vi "Ex2_Adquiere_Datos.vi"(8 "error in (no error)":errorcluster, 11 "LINX Resource in":T2) -> (0 "error out":errorcluster, 2 "Señales":T1, 3 "LINX Resource out":T2)   [LabVIEW 2020]
uses:
  <vilib>/MakerHub/LINX/Private/Type Defs/LINX Ref.ctl
  <vilib>/MakerHub/LINX/Private/Type Defs/Platform.ctl
  <vilib>/MakerHub/LINX/Private/Type Defs/Interface.ctl
  <vilib>/MakerHub/LINX/Private/Device/Type Defs/LINX Device Config.ctl
  <vilib>/MakerHub/LINX/Private/Device/Type Defs/TCP Config.ctl
  <vilib>/MakerHub/LINX/Private/Device/Type Defs/Channels.ctl
  <vilib>/MakerHub/LINX/Public/Peripherals/Analog/Analog Read N Chans.vi
  <vilib>/MakerHub/LINX/Public/Peripherals/Digital/Digital Read N Chans.vi
  <vilib>/MakerHub/LINX/Private/Local IO/LinxAnalogRead.vi
  <vilib>/MakerHub/LINX/Public/Utilities/Check Channel.vi
  <vilib>/MakerHub/LINX/Private/Local IO/LinxDigitalRead.vi
  <vilib>/MakerHub/LINX/Private/Utilties/Generate Error.vi
  <vilib>/MakerHub/LINX/LMH-LINX.lvlib
  <vilib>/MakerHub/LINX/Private/Device/Device.lvlib
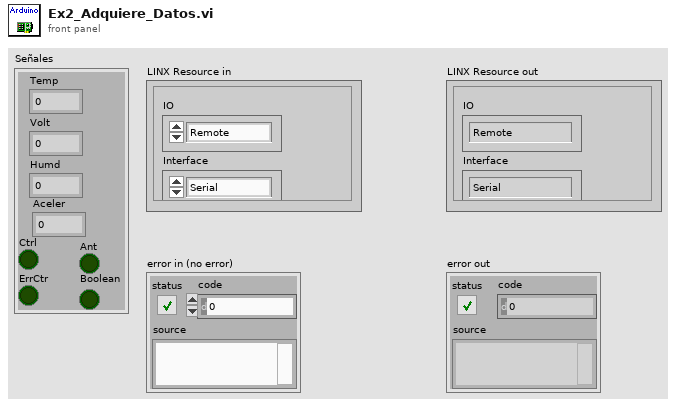
[diagram p1: front panel]
types:
  T1 = cluster{"Temp":dbl, "Volt":dbl, "Humd":dbl, "Ant":bool, "Ctrl":bool, "ErrCtr":bool, "Aceler":dbl, "Boolean":bool}
  T2 = typedef "LMH-LINX.lvlib/LINX Ref.ctl" = cluster{"IO":T3, "Interface":T4, "LINX Device Config":T5}
  T3 = typedef "LMH-LINX.lvlib/Platform.ctl" = enum16{"Remote", "Local"}
  T4 = typedef "LMH-LINX.lvlib/Interface.ctl" = enum16{"Serial", "TCP"}
  T5 = typedef "LMH-LINX.lvlib/Device.lvlib/LINX Device Config.ctl" = cluster{"Interface":T4, "COM Port":refnum<visa-resource-name>, "TCP Configuration":T6, "Device Family":u8, "Device ID":u8, "Device Name":string, "TCP Ref":refnum<k5>, "Channels":T7}
  T6 = typedef "LMH-LINX.lvlib/Device.lvlib/TCP Config.ctl" = cluster{"IP Address":string, "Port":u16}
  T7 = typedef "LMH-LINX.lvlib/Channels.ctl" = cluster{"DI":u8[], "DO":u8[], "AI":u8[], "AO":u8[], "PWM":u8[], "QE":u8[], "UART":u8[], "I2C 2":u8[], "SPI":u8[], "CAN":u8[], "Servo":u8[], "AI Ref (V)":dbl, "AI Resolution (Bits)":u8, "AO Ref (V)":dbl, "AO Resolution (Bits)":u8}
  T8 = cluster{"Temp":dbl, "Volt":dbl, "Humd":dbl, "Ant":bool, "Ctrl":bool, "ErrCtr":bool, "Aceler":dbl, "Sts_Tx-Rx":bool}
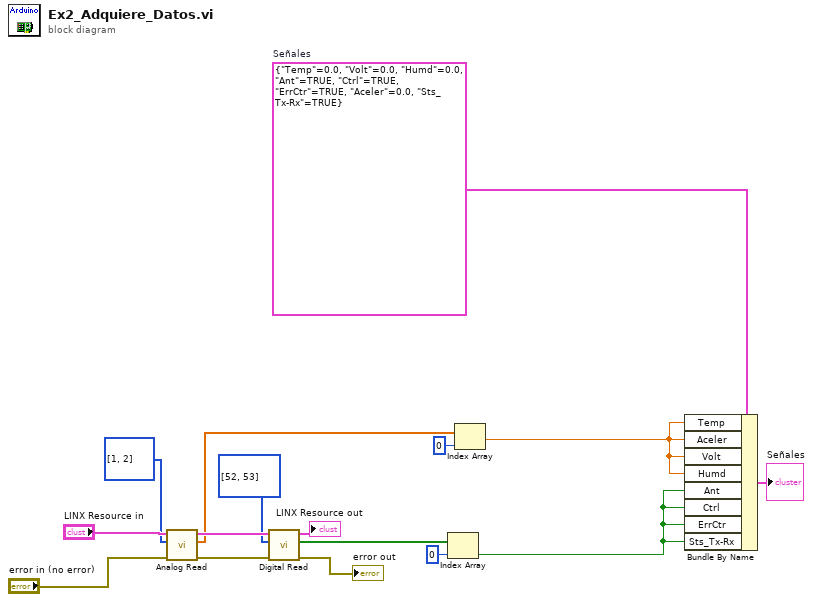
[diagram p0: block diagram]
diagram:
  w15 = T8 {"Temp"=0.0, "Volt"=0.0, "Humd"=0.0, "Ant"=TRUE, "Ctrl"=TRUE, "ErrCtr"=TRUE, "Aceler"=0.0, "Sts_Tx-Rx"=TRUE}  # Señales
  n1 = call-poly <vilib>:"Analog Read.vi"("Error In"="error in (no error)", "AI Channel(s)"=u8[] [1, 2], "LINX Resource"="LINX Resource in") -> ("Error Out"=w9:errorcluster, "Voltages"=w4:dbl[], "LINX Resource"=w12:T2)  [unwired: 5 in, 1 out]
  n2 = call-poly <vilib>:"Digital Read.vi"("Error In"=w9, "DI Channels"=u8[] [52, 53], "LINX Resource"=w12) -> ("Error Out"=→"error out":errorcluster, "Values"=w3:bool[], "LINX Resource"=→"LINX Resource out":T2)  [unwired: 6 in]
  n3 = Index Array(array=w3, index=0) -> (element=w1:bool)
  n4 = Index Array(array=w4, index=0) -> (element=w6:dbl)
  n5 = Bundle By Name(cluster=w15, "Temp"=w6, "Aceler"=w6, "Volt"=w6, "Humd"=w6, "Ant"=w1, "Ctrl"=w1, "ErrCtr"=w1, "Sts_Tx-Rx"=w1) -> (→"Señales":T8)
